vi "Sort by Time.vi"(11 "Sheet Array":string[][](array[string])=[["Horse", "1", "2"], ["Monkey", "100", "200"], ["elephant", "1000", "2000"], ["chicken", "10000", "20000"]]) -> (3 "sorted array":string[][](array[string]))   [LabVIEW 2015]
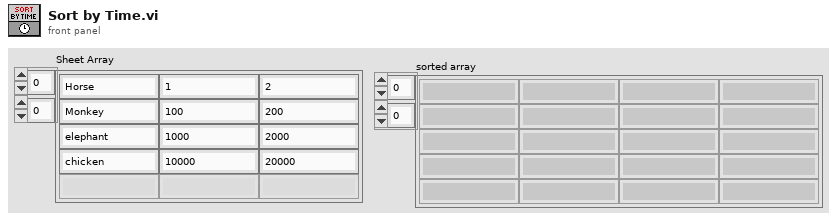
[diagram p1: front panel]
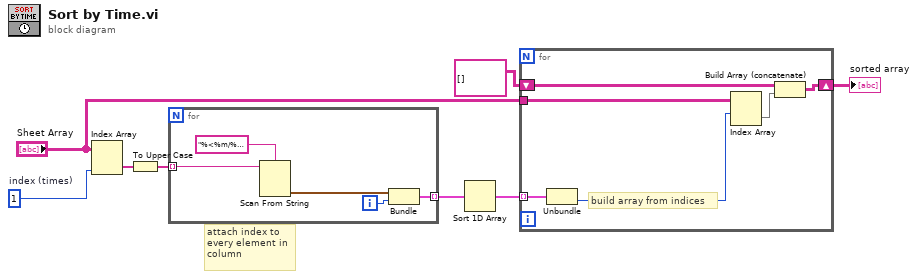
[diagram p0: block diagram]
diagram:
  w1 = 1  # index (times)
  # "attach index to \nevery element in\ncolumn"
  n1 = Index Array(array="Sheet Array", index (col)=w1) -> (element=w4:string[])  [unwired: 1 in]
  n2 = To Upper Case(1:w4) -> (0:w3:string[])
  n3 = for {
    tunnel: w3 -> [w10] mode=indexing
    tunnel: [w12] -> w8 mode=indexing
    i -> [w13]
    n4 = Scan From String "Scan From String"(format string="%<%m/%d/%Y %I:%M:%S%3u %p>T", input string=w10) -> (output 1=w9:timestamp)  [unwired: 3 in, 3 out]
    n5 = Bundle(w9, w13) -> (w12:cluster{timestamp, i32})  [unwired: 1 in]
  }
  n6 = Sort 1D Array(array=w8) -> (sorted array=w5:cluster{timestamp, i32}[])
  n7 = for {
    tunnel: "Sheet Array" -> [w17]
    shift-right: [w15] -> w2
    shift-left: string[][] [] ("Array") -> [w16]
    tunnel: w5 -> [w19] mode=indexing
    # "build array from indices"
    n8 = Unbundle(w19) -> (w18:i32)  [unwired: 1 out]
    n9 = Index Array(array=w17, index (row)=w18) -> (element=w14:string[])  [unwired: 1 in]
    n10 = Build Array (concatenate)(w16, w14) -> (w15:string[][])
  }
  "sorted array" <- w2
